vi "USBShutdown.vi"(8 "error in (no error)":errorcluster, 11 "USBLib In":refnum<k24>) -> (0 "error out":errorcluster)   [LabVIEW 2009]
uses:
  C:/Samples/LabVIEW/UseDeviceKey/LabVIEW 2009/UseDeviceKey (with Device VIs)/UsbDllWrap.dll
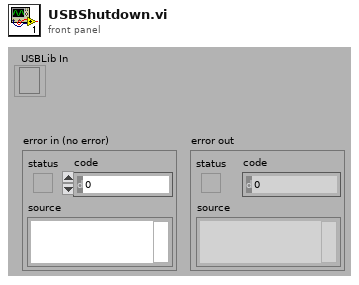
[diagram p1: front panel]
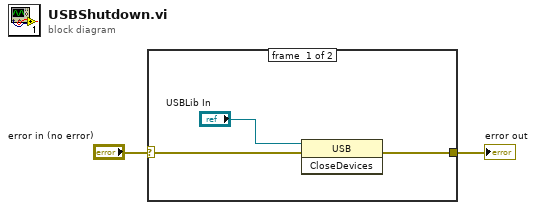
[diagram p0: block diagram]
diagram:
  n1 = case shown="No Error" "error in (no error)" {
    selector: "error in (no error)" -> [w4 w6]
    tunnel: [w3 w6] -> w1
    frame #0 {
      n2 = invoke class="USB" method="CloseDevices"(reference="USBLib In", error in=w4) -> (error out=w3:errorcluster)  [unwired: 1 in, 2 out]
    }
    frame #1 {
    }
  }
  "error out" <- w1
